vi "StringToDBL(cast).vi"(1 "String":string) -> (0 "DBL":dbl)   [LabVIEW 2012]
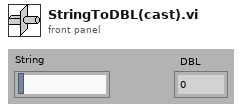
[diagram p1: front panel]
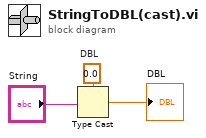
[diagram p0: block diagram]
diagram:
  w2 = 0.0  # DBL
  n1 = Type Cast(type=w2, x="String") -> (*(type *) &x=→"DBL":dbl)
